vi "FPGA Read Indicator Array Address by Index.vi"(8 "error in (no error)":errorcluster, 9 "index":i32, 10 "Data Type":T1, 11 "FPGA Interface Base in":refnum<class "FPGA Interface Base.lvclass">) -> (0 "error out":errorcluster, 1 "Found?":bool, 2 "Address":u32, 3 "FPGA Interface Base out":refnum<class "FPGA Interface Base.lvclass">, 5 "Num Elements":u32)   [LabVIEW 2010, in "FPGA Interface Base.lvclass"]
uses:
  <userlib>/_FPGA Interface Advanced Tools/FPGA Interface Base/FPGA Interface Base.lvclass
  <vilib>/rvi/DataTransferAndStorage/Container/Common/niFpgaDataTypeControl.ctl
  <userlib>/_FPGA Interface Advanced Tools/FPGA Interface Base/FPGA Interface Base.lvclass/FPGA Interface Base.ctl
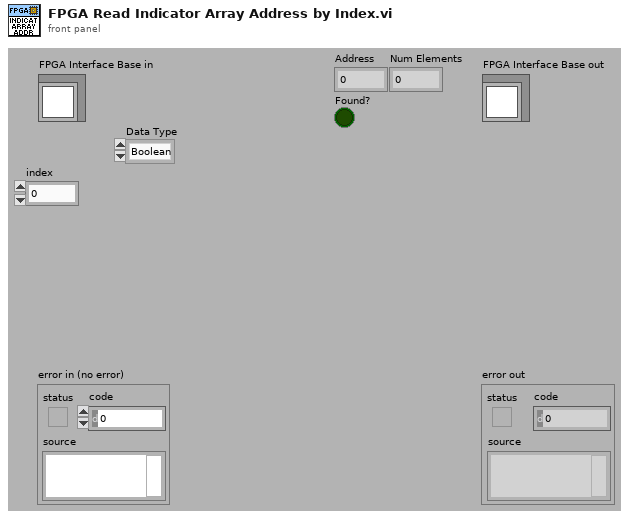
[diagram p1: front panel]
types:
  T1 = typedef "niFpgaDataTypeControl.ctl" = enum32{"Boolean", "I8", "I16", "I32", "I64", "U8", "U16", "U32", "U64", "FXP", "CustomControl"}
  T2 = typedef "FPGA Interface Base.lvclass/FPGA Session.ctl" = refnum<data-value>
  T3 = typedef "FPGA Interface Base.lvclass/FPGA Session Data.ctl" = cluster{"Session Out":u32, "Indicator Scalars":T4, "Indicator Arrays":T6, "Control Scalars":T4, "Control Arrays":T6, "TargetToHost FIFO Channels":T8, "HostToTarget FIFO Channels":T8, "All FIFOs":T9[], "IRQ Context Queue":refnum<queue>}
  T4 = typedef "FPGA Bitfile Utility.lvlib/Scalar Register Set.ctl" = cluster{"Boolean":T5[], "I8":T5[], "I16":T5[], "I32":T5[], "I64":T5[], "U8":T5[], "U16":T5[], "U32":T5[], "U64":T5[]}
  T5 = typedef "FPGA Bitfile Utility.lvlib/Scalar Register.ctl" = cluster{"Address":u32, "Name":string}
  T6 = typedef "FPGA Bitfile Utility.lvlib/Array Register Set.ctl" = cluster{"Boolean":T7[], "I8":T7[], "I16":T7[], "I32":T7[], "I64":T7[], "U8":T7[], "U16":T7[], "U32":T7[], "U64":T7[]}
  T7 = typedef "FPGA Bitfile Utility.lvlib/Array Register.ctl" = cluster{"Address":u32, "Num Elements":u32, "Name":string}
  T8 = typedef "FPGA Bitfile Utility.lvlib/FIFO Channel Set.ctl" = cluster{"Boolean":T9[], "I8":T9[], "I16":T9[], "I32":T9[], "I64":T9[], "U8":T9[], "U16":T9[], "U32":T9[], "U64":T9[]}
  T9 = typedef "FPGA Bitfile Utility.lvlib/FIFO Channel.ctl" = cluster{"Physical Channel":u32, "Name":string}
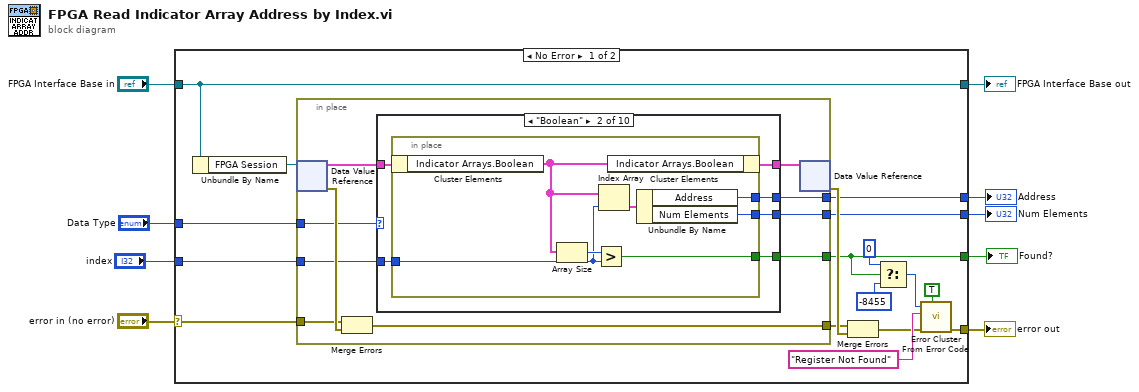
[diagram p0: block diagram]
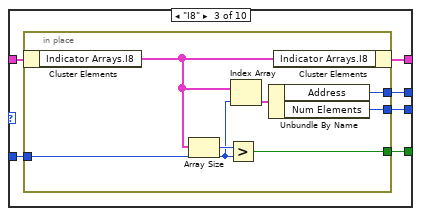
[diagram p3: hidden frame]
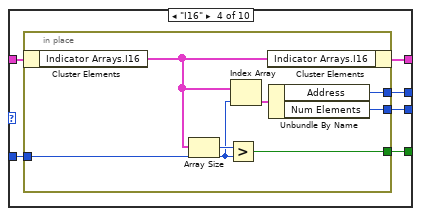
[diagram p4: hidden frame]
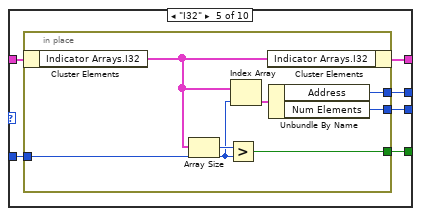
[diagram p5: hidden frame]
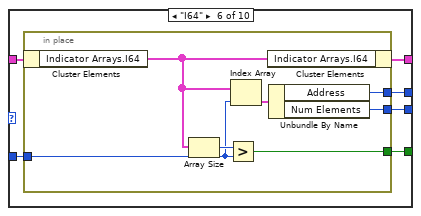
[diagram p6: hidden frame]
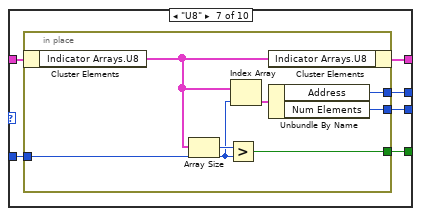
[diagram p7: hidden frame]
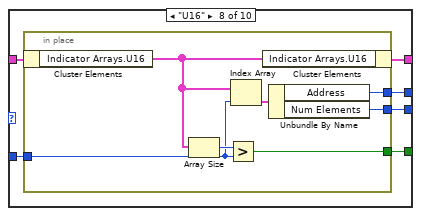
[diagram p8: hidden frame]
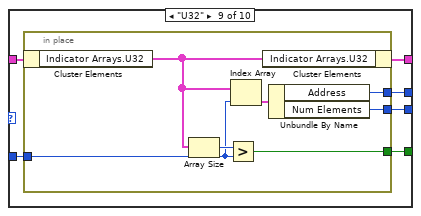
[diagram p9: hidden frame]
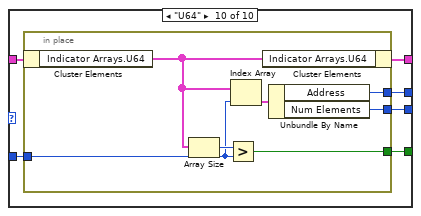
[diagram p10: hidden frame]
diagram:
  n1 = case shown="No Error" "error in (no error)" {
    selector: "error in (no error)" -> [w21 w155]
    tunnel: [w12 w155] -> w8
    tunnel: [w26 w156] -> w6
    tunnel: "FPGA Interface Base in" -> [w26 w156]
    tunnel: [w22 _] -> w5
    tunnel: [w10 _] -> w4
    tunnel: "Data Type" -> [w20 _]
    tunnel: "index" -> [w19 _]
    tunnel: [w18 _] -> w1
    frame No Error {
      n2 = Unbundle By Name(w26) -> ("FPGA Session"=w23:T2)
      n3 = in-place {
        in-place-border: [w33] -> w22
        in-place-border: [w32] -> w10
        in-place-border: [w31] -> w24
        in-place-border: w21 -> [w30]
        in-place-border: w20 -> [w29]
        in-place-border: w19 -> [w28]
        in-place-border: [w27] -> w18
        n4 = in-place-dvr #1(w23) -> (w35:T3, w36:errorcluster)
        n5 = Merge Errors(w30, w36) -> (w31:errorcluster)
        n6 = case shown="\"Boolean\"" w29 {
          tunnel: w35 -> [w37 w43 w56 w69 w82 w95 w108 w121 w134 w147]
          tunnel: [w37 w42 w55 w68 w81 w94 w107 w120 w133 w146] -> w34
          tunnel: [_ w41 w54 w67 w80 w93 w106 w119 w132 w145] -> w33
          tunnel: [_ w40 w53 w66 w79 w92 w105 w118 w131 w144] -> w32
          tunnel: w28 -> [_ w39 w52 w65 w78 w91 w104 w117 w130 w143]
          tunnel: [_ w38 w51 w64 w77 w90 w103 w116 w129 w142] -> w27
          frame Default {
          }
          frame "Boolean" {
            n7 = in-place {
              in-place-border: [w50] -> w41
              in-place-border: [w48] -> w40
              in-place-border: w39 -> [w45]
              in-place-border: [w44] -> w38
              n8 = in-place-cluster #2(w43) -> ("Indicator Arrays.Boolean"=w47:T7[])
              n9 = Array Size(array=w47) -> (size(s)=w49:i32)
              n10 = Greater?(x=w49, y=w45) -> (0:w48:bool)
              n11 = Index Array(array=w47, index=w45) -> (element=w46:T7)
              n12 = in-place-cluster #2("Indicator Arrays.Boolean"=w47) -> (w42:T3)
              n13 = Unbundle By Name(w46) -> ("Address"=w50:u32, "Num Elements"=w44:u32)
            }
          }
          frame "I8" {
            n14 = in-place {
              in-place-border: [w63] -> w54
              in-place-border: [w61] -> w53
              in-place-border: w52 -> [w58]
              in-place-border: [w57] -> w51
              n15 = in-place-cluster #3(w56) -> ("Indicator Arrays.I8"=w60:T7[])
              n16 = Array Size(array=w60) -> (size(s)=w62:i32)
              n17 = Greater?(x=w62, y=w58) -> (0:w61:bool)
              n18 = Index Array(array=w60, index=w58) -> (element=w59:T7)
              n19 = Unbundle By Name(w59) -> ("Address"=w63:u32, "Num Elements"=w57:u32)
              n20 = in-place-cluster #3("Indicator Arrays.I8"=w60) -> (w55:T3)
            }
          }
          frame "I16" {
            n21 = in-place {
              in-place-border: [w76] -> w67
              in-place-border: [w74] -> w66
              in-place-border: w65 -> [w71]
              in-place-border: [w70] -> w64
              n22 = in-place-cluster #4(w69) -> ("Indicator Arrays.I16"=w73:T7[])
              n23 = Array Size(array=w73) -> (size(s)=w75:i32)
              n24 = Greater?(x=w75, y=w71) -> (0:w74:bool)
              n25 = Index Array(array=w73, index=w71) -> (element=w72:T7)
              n26 = in-place-cluster #4("Indicator Arrays.I16"=w73) -> (w68:T3)
              n27 = Unbundle By Name(w72) -> ("Address"=w76:u32, "Num Elements"=w70:u32)
            }
          }
          frame "I32" {
            n28 = in-place {
              in-place-border: [w89] -> w80
              in-place-border: [w87] -> w79
              in-place-border: w78 -> [w84]
              in-place-border: [w83] -> w77
              n29 = in-place-cluster #5(w82) -> ("Indicator Arrays.I32"=w86:T7[])
              n30 = Array Size(array=w86) -> (size(s)=w88:i32)
              n31 = Greater?(x=w88, y=w84) -> (0:w87:bool)
              n32 = Index Array(array=w86, index=w84) -> (element=w85:T7)
              n33 = in-place-cluster #5("Indicator Arrays.I32"=w86) -> (w81:T3)
              n34 = Unbundle By Name(w85) -> ("Address"=w89:u32, "Num Elements"=w83:u32)
            }
          }
          frame "I64" {
            n35 = in-place {
              in-place-border: [w102] -> w93
              in-place-border: [w100] -> w92
              in-place-border: w91 -> [w97]
              in-place-border: [w96] -> w90
              n36 = in-place-cluster #6(w95) -> ("Indicator Arrays.I64"=w99:T7[])
              n37 = Array Size(array=w99) -> (size(s)=w101:i32)
              n38 = Greater?(x=w101, y=w97) -> (0:w100:bool)
              n39 = Index Array(array=w99, index=w97) -> (element=w98:T7)
              n40 = in-place-cluster #6("Indicator Arrays.I64"=w99) -> (w94:T3)
              n41 = Unbundle By Name(w98) -> ("Address"=w102:u32, "Num Elements"=w96:u32)
            }
          }
          frame "U8" {
            n42 = in-place {
              in-place-border: [w115] -> w106
              in-place-border: [w113] -> w105
              in-place-border: w104 -> [w110]
              in-place-border: [w109] -> w103
              n43 = in-place-cluster #7(w108) -> ("Indicator Arrays.U8"=w112:T7[])
              n44 = Array Size(array=w112) -> (size(s)=w114:i32)
              n45 = Greater?(x=w114, y=w110) -> (0:w113:bool)
              n46 = Index Array(array=w112, index=w110) -> (element=w111:T7)
              n47 = in-place-cluster #7("Indicator Arrays.U8"=w112) -> (w107:T3)
              n48 = Unbundle By Name(w111) -> ("Address"=w115:u32, "Num Elements"=w109:u32)
            }
          }
          frame "U16" {
            n49 = in-place {
              in-place-border: [w128] -> w119
              in-place-border: [w126] -> w118
              in-place-border: w117 -> [w123]
              in-place-border: [w122] -> w116
              n50 = in-place-cluster #8(w121) -> ("Indicator Arrays.U16"=w125:T7[])
              n51 = Array Size(array=w125) -> (size(s)=w127:i32)
              n52 = Greater?(x=w127, y=w123) -> (0:w126:bool)
              n53 = Index Array(array=w125, index=w123) -> (element=w124:T7)
              n54 = in-place-cluster #8("Indicator Arrays.U16"=w125) -> (w120:T3)
              n55 = Unbundle By Name(w124) -> ("Address"=w128:u32, "Num Elements"=w122:u32)
            }
          }
          frame "U32" {
            n56 = in-place {
              in-place-border: [w141] -> w132
              in-place-border: [w139] -> w131
              in-place-border: w130 -> [w136]
              in-place-border: [w135] -> w129
              n57 = in-place-cluster #9(w134) -> ("Indicator Arrays.U32"=w138:T7[])
              n58 = Array Size(array=w138) -> (size(s)=w140:i32)
              n59 = Greater?(x=w140, y=w136) -> (0:w139:bool)
              n60 = Index Array(array=w138, index=w136) -> (element=w137:T7)
              n61 = in-place-cluster #9("Indicator Arrays.U32"=w138) -> (w133:T3)
              n62 = Unbundle By Name(w137) -> ("Address"=w141:u32, "Num Elements"=w135:u32)
            }
          }
          frame "U64" {
            n63 = in-place {
              in-place-border: [w154] -> w145
              in-place-border: [w152] -> w144
              in-place-border: w143 -> [w149]
              in-place-border: [w148] -> w142
              n64 = in-place-cluster #10(w147) -> ("Indicator Arrays.U64"=w151:T7[])
              n65 = Array Size(array=w151) -> (size(s)=w153:i32)
              n66 = Greater?(x=w153, y=w149) -> (0:w152:bool)
              n67 = Index Array(array=w151, index=w149) -> (element=w150:T7)
              n68 = in-place-cluster #10("Indicator Arrays.U64"=w151) -> (w146:T3)
              n69 = Unbundle By Name(w150) -> ("Address"=w154:u32, "Num Elements"=w148:u32)
            }
          }
        }
        n70 = in-place-dvr #1(w34) -> (w25:errorcluster)  [unwired: 1 out]
      }
      n71 = Merge Errors(w24, w25) -> (w11:errorcluster)
      n72 = Select(t=0, s=w10, f=-8455 ("error code (0)")) -> (s? t:f=w14:i32)
      n73 = call <vilib>:"Error Cluster From Error Code.vi"("show call chain? (False)"=TRUE, "error in (no error)"=w11, "error message (\"\")"="Register Not Found" ("string"), "error code (0)"=w14) -> ("error out"=w12:errorcluster)  [unwired: 5 in]
    }
    frame Error {
    }
  }
  "error out" <- w8
  "FPGA Interface Base out" <- w6
  "Address" <- w5
  "Found?" <- w4
  "Num Elements" <- w1
